vi "Set Read Position.vi"(8 "error in (no error)":errorcluster, 10 "Read Position":i64, 11 "FileStream in":refnum<class "FileStream.lvclass">) -> (0 "error out":errorcluster, 3 "FileStream out":refnum<class "FileStream.lvclass">)   [LabVIEW 2020, in "Stream.lvlib" / "FileStream.lvclass"]
uses:
  FileStream.lvclass
  FileStream.lvclass/FileStream.ctl
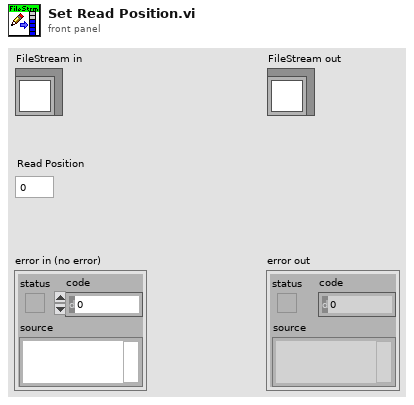
[diagram p1: front panel]
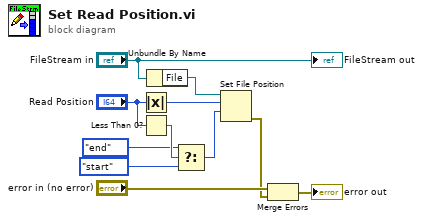
[diagram p0: block diagram]
diagram:
  n1 = Absolute Value(x="Read Position") -> (abs(x)=w7:i64)
  n2 = Less Than 0?(x="Read Position") -> (x < 0?=w6:bool)
  n3 = Unbundle By Name("FileStream in") -> ("File"=w9:refnum<file>)
  n4 = Select(t=enum16{"start", "end", "current"}."end" ("from (0:start)"), s=w6, f=enum16{"start", "end", "current"}."start" ("from (0:start)")) -> (s? t:f=w3:enum16{"start", "end", "current"})
  n5 = Set File Position(offset (in bytes) (0)=w7, refnum=w9, from (0:start)=w3) -> (error out=w1:errorcluster)  [unwired: 1 in, 1 out]
  n6 = Merge Errors("error in (no error)", w1) -> (→"error out":errorcluster)
  "FileStream out" <- "FileStream in"
